vi "SetVisionFPS.vi"(8 "error in (no error)":errorcluster, 9 "tempo UDP":dbl format="%#_13g", 10 "tempo Vision":dbl format="%#_13g", 11 "Vision in":refnum<class "Vision.lvclass">) -> (0 "error out":errorcluster, 2 "milliseconds to wait":dbl, 3 "Vision out":refnum<class "Vision.lvclass">)   [LabVIEW 2020, in "Vision.lvclass"]
uses:
  Vision.lvclass
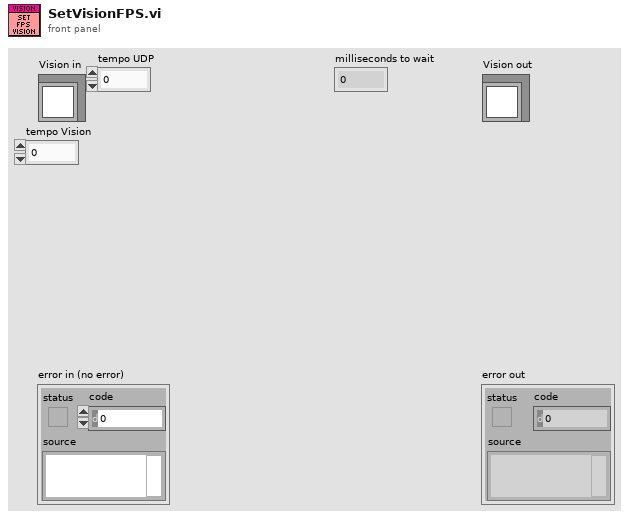
[diagram p1: front panel]
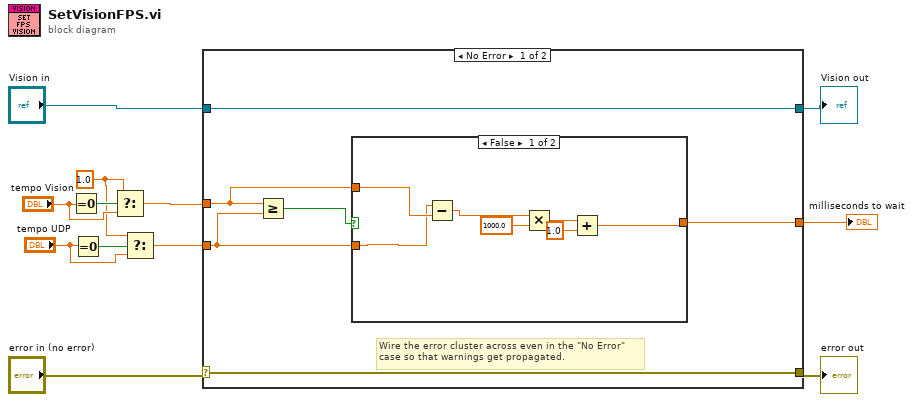
[diagram p0: block diagram]
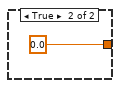
[diagram p2: hidden frame]
diagram:
  w3 = 1.0 ("t")
  n1 = Equal To 0?(x="tempo Vision") -> (x = 0?=w6:bool)
  n2 = Equal To 0?(x="tempo UDP") -> (x = 0?=w7:bool)
  n3 = Select(t=w3, s=w6, f="tempo Vision") -> (s? t:f=w1:dbl)
  n4 = Select(t=w3, s=w7, f="tempo UDP") -> (s? t:f=w2:dbl)
  n5 = case shown="No Error" "error in (no error)" {
    selector: "error in (no error)" -> [w17 w28]
    tunnel: [w17 w28] -> w11
    tunnel: [w18 w27] -> w9
    tunnel: "Vision in" -> [w18 w27]
    tunnel: w1 -> [w14 _]
    tunnel: w2 -> [w13 _]
    tunnel: [w15 _] -> w8
    frame No Error {
      # "Wire the error cluster across even in the \"No Error\"\ncase so that warnings get propagated."
      n6 = Greater Or Equal?(x=w14, y=w13) -> (x >= y?=w16:bool)
      n7 = case shown="False" w16 {
        tunnel: [w19 0.0] -> w15
        tunnel: w14 -> [w23 _]
        tunnel: w13 -> [w22 _]
        frame False {
          n8 = Subtract(x=w22, y=w23) -> (x-y=w25:dbl)
          n9 = Multiply(x=w25, y=1000.0) -> (x*y=w21:dbl)
          n10 = Add(x=w21, y=1.0) -> (x+y=w19:dbl)
        }
        frame True {
        }
      }
    }
    frame Error {
    }
  }
  "error out" <- w11
  "Vision out" <- w9
  "milliseconds to wait" <- w8
